vi "Log Error.vi"(8 "error in (no error)":errorcluster, 11 "Logger.Error in":refnum<class "Logger.Error.lvclass">) -> (0 "error out":errorcluster, 3 "Logger.Error out":refnum<class "Logger.Error.lvclass">)   [LabVIEW 2016, in "Logger.Error.lvclass"]
uses:
  Logger.Error.lvclass
  <userlib>/_MGI/Error Reporter/MGI Error Reporter Base/MGI Error Reporter Base.lvclass
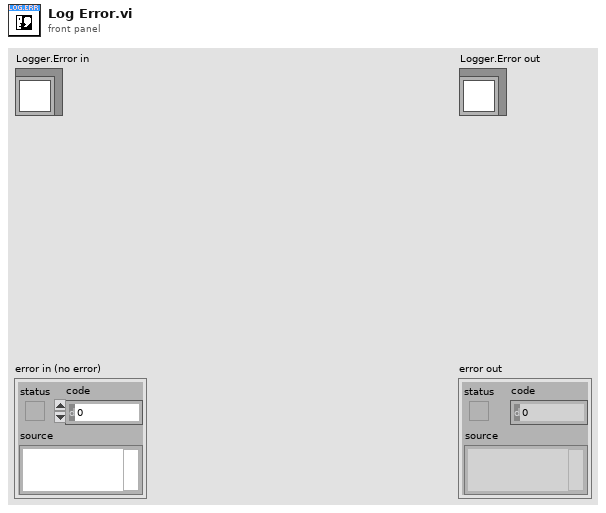
[diagram p1: front panel]
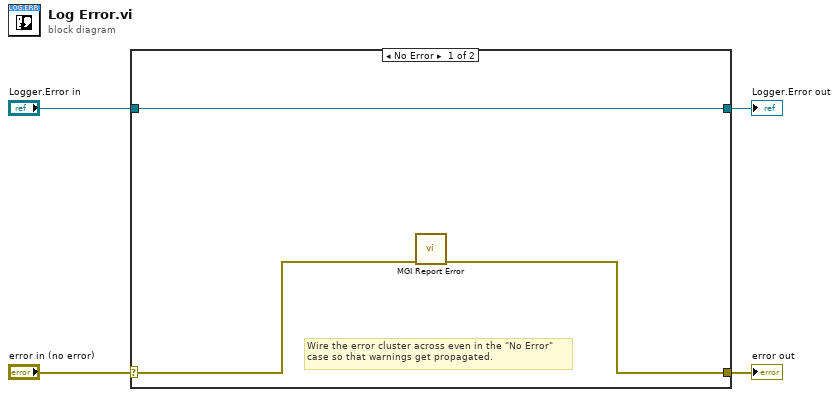
[diagram p0: block diagram]
diagram:
  n1 = case shown="No Error" "error in (no error)" {
    selector: "error in (no error)" -> [w6 w9]
    tunnel: [w5 w9] -> w3
    tunnel: [w7 w8] -> w1
    tunnel: "Logger.Error in" -> [w7 w8]
    frame No Error {
      # "Wire the error cluster across even in the \"No Error\"\ncase so that warnings get propagated."
      n2 = call <userlib>:"MGI Report Error.vi"("error in"=w6) -> ("no error"=w5:errorcluster)  [unwired: 10 in]
    }
    frame Error {
    }
  }
  "error out" <- w3
  "Logger.Error out" <- w1
